vi "Merge Maps.vi"(9 "Secondary Map":variant, 10 "Primary Map":variant) -> (2 "Merged Map":variant)   [LabVIEW 2013]
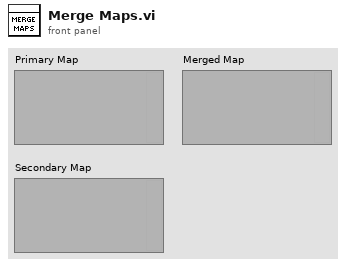
[diagram p1: front panel]
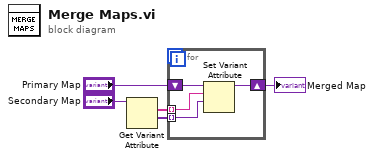
[diagram p0: block diagram]
diagram:
  n1 = Get Variant Attribute(Variant="Secondary Map") -> (names=w3:string[], values=w2:variant[])  [unwired: 3 in, 2 out]
  n2 = for {
    shift-right: [w8] -> w1
    shift-left: "Primary Map" -> [w9]
    tunnel: w3 -> [w7] mode=indexing
    tunnel: w2 -> [w6] mode=indexing
    n3 = Set Variant Attribute(Variant=w9, name=w7, value=w6) -> (Variant out=w8:variant)  [unwired: 1 in, 2 out]
  }
  "Merged Map" <- w1
